vi "ViewContact.vi"(7 "LabVIEW Web Service Request":refnum<class "Web Request.lvclass">, 9 "uuid":string, 10 "Edit":bool, 11 "ID":u32) -> ()   [LabVIEW 2014]
doc: "This HTTP Method VI shows an existing contact and optionally provides a form for editing the contact information."
uses:
  <vilib>/wsapi/Web Request.lvclass
  <vilib>/wsapi/class/subVIs/Set String ESP Variable.vi
panel:
  # "Because this is an HTTP Method VI, LabVIEW Web Service Request is populated automatically."
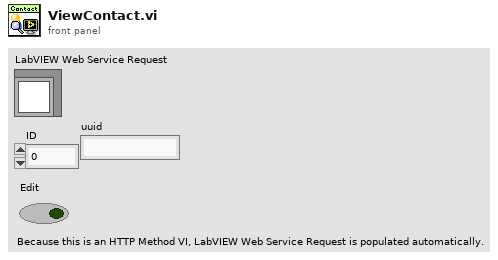
[diagram p1: front panel]
types:
  T1 = cluster{"train_data":cluster{"uuid":string, "int":i32, "posit_array":cluster{"x":dbl, "y":dbl, "z":dbl}[]}, "train_control":cluster{"uuid":string, "throttle":dbl, "brake":dbl, "horn":dbl, "wait":dbl, "name":string, "mode":string, "dest":string}}
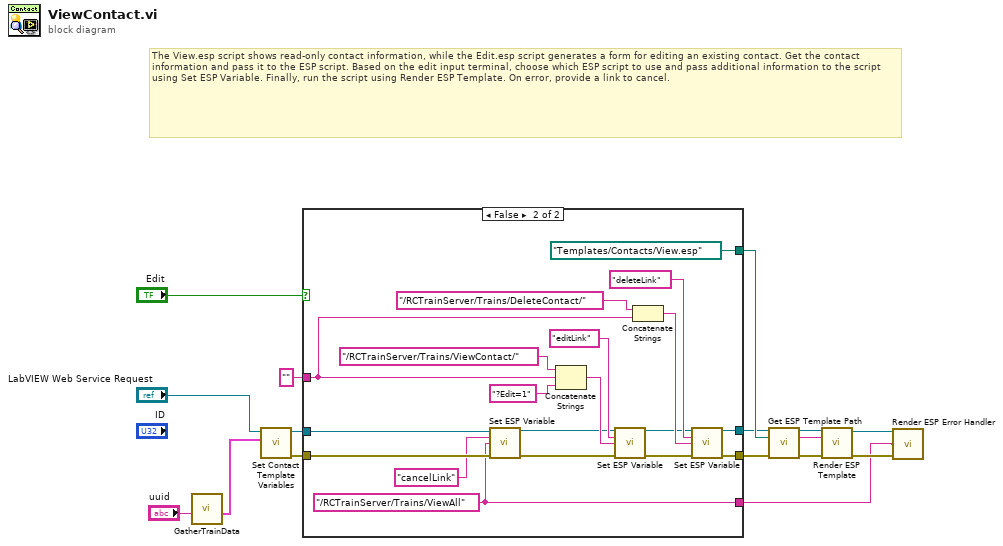
[diagram p0: block diagram]
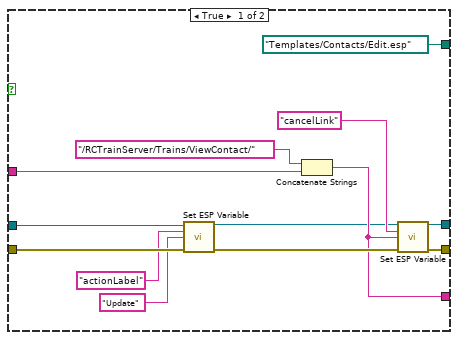
[diagram p2: hidden frame]
diagram:
  # "The View.esp script shows read-only contact information, while the Edit.esp script generates a form for editing an existing contact. Get the contact information and pass it to the ESP script. Based on the edit input terminal, choose which ESP script to use and pass additional information to the script using Set ESP Variable. Finally, run the script using Render ESP Template. On error, provide a link to cancel."
  n1 = call "GatherTrainData.vi"("uuid"="uuid") -> ("Cluster"=w3:T1)  [unwired: 8 in, 2 out]
  n2 = call "Set Contact Template Variables.vi"("Cluster"=w3, "LabVIEW Web Service Request"="LabVIEW Web Service Request") -> ("error out"=w14:errorcluster, "LabVIEW Web Service Request out"=w13:refnum<class "Web Request.lvclass">)  [unwired: 8 in]
  n3 = case shown="False" "Edit" {
    tunnel: [path "Templates/Contacts/Edit.esp" path "Templates/Contacts/View.esp"] -> w12
    tunnel: w13 -> [w17 w31]
    tunnel: w14 -> [w29 w48]
    tunnel: [w25 w43] -> w4
    tunnel: [w24 w42] -> w11
    tunnel: "" -> [w21 w36]
    tunnel: [w19 w34] -> w6
    frame True {
      n4 = call-poly <vilib>:"Set ESP Variable.vi"("LabVIEW Web Service Request"=w17, "key"="actionLabel", "value"="Update", "error in (no error)"=w29) -> ("LabVIEW Web Service Request out"=w18:refnum<class "Web Request.lvclass">, "error out"=w26:errorcluster)  [unwired: 10 in]
      n5 = Concatenate Strings("/RCTrainServer/Trains/ViewContact/" ("value"), w21) -> (w19:string)
      n6 = call-poly <vilib>:"Set ESP Variable.vi"("LabVIEW Web Service Request"=w18, "key"="cancelLink", "value"=w19, "error in (no error)"=w26) -> ("LabVIEW Web Service Request out"=w25:refnum<class "Web Request.lvclass">, "error out"=w24:errorcluster)  [unwired: 10 in]
    }
    frame False {
      w34 = "/RCTrainServer/Trains/ViewAll" ("value")
      n7 = call-poly <vilib>:"Set ESP Variable.vi"("LabVIEW Web Service Request"=w31, "key"="cancelLink", "value"=w34, "error in (no error)"=w48) -> ("LabVIEW Web Service Request out"=w32:refnum<class "Web Request.lvclass">, "error out"=w46:errorcluster)  [unwired: 10 in]
      n8 = Concatenate Strings("/RCTrainServer/Trains/ViewContact/" ("value"), w36, "?Edit=1" ("string")) -> (w37:string)
      n9 = call-poly <vilib>:"Set ESP Variable.vi"("LabVIEW Web Service Request"=w32, "key"="editLink", "value"=w37, "error in (no error)"=w46) -> ("LabVIEW Web Service Request out"=w30:refnum<class "Web Request.lvclass">, "error out"=w44:errorcluster)  [unwired: 10 in]
      n10 = Concatenate Strings("/RCTrainServer/Trains/DeleteContact/" ("value"), w36) -> (w38:string)
      n11 = call-poly <vilib>:"Set ESP Variable.vi"("LabVIEW Web Service Request"=w30, "key"="deleteLink", "value"=w38, "error in (no error)"=w44) -> ("LabVIEW Web Service Request out"=w43:refnum<class "Web Request.lvclass">, "error out"=w42:errorcluster)  [unwired: 10 in]
    }
  }
  n12 = call "Get ESP Template Path.vi"("LabVIEW Web Service Request"=w4, "Relative Template Path"=w12, "error in (no error)"=w11) -> ("LabVIEW Web Service Request out"=w5:refnum<class "Web Request.lvclass">, "Template Name"=w7:string, "error out"=w10:errorcluster)  [unwired: 10 in]
  n13 = call <vilib>:"Render ESP Template.vi"("LabVIEW Web Service Request"=w5, "espName"=w7, "error in (no error)"=w10) -> ("LabVIEW Web Service Request out"=w8:refnum<class "Web Request.lvclass">, "error out"=w9:errorcluster)  [unwired: 11 in]
  n14 = call "Render ESP Error Handler.vi"("LabVIEW Web Service Request"=w8, "Link"=w6, "error in (no error)"=w9) -> ()  [unwired: 11 in, 2 out]
